vi "WT500 Get Power Data.vi"(7 "Error In":errorcluster, 10 "VISA resource name":refnum<visa-resource-name>) -> (0 "Error Out":errorcluster, 1 "Power Data Out":T1={"Current (A):Element 1"=236.2, "Current (A):Element 2"=17.749, "Power (W):Sigma"=4192.0, "Watt Hours (Wh):Sigma"=0.0, "Voltage (V):Element 2"=236.2, "Voltage (V):Element 1"=236.2, "Current Crest Factor:Element 1"=0.0, "Current Crest Factor:Element 2"=0.0, "Voltage Harmonic (%):Element 1"=0.0, "Voltage Harmonic (%):Element 2"=0.0, "Voltage Crest Factor:Element 1"=0.0, "Voltage Crest Factor:Element 2"=0.0, "Time:Element 1"=0.0, "Frequency (Hz):Element 1"=0.0, "Apparent Power (VA):Element 1"=0.0, "Apparent Power (VA):Element 2"=0.0, "Power Factor:Element 1"=0.0, "Power Factor:Element 2"=0.0, "Max Watt Hours"=0.0, "Voltage (V):Element 2 Avg"=0.0, "Voltage (V):Element 1 Avg"=0.0} {"Voltage (V):Element 1 Avg" format="%.3g"; "Voltage (V):Element 2 Avg" format="%.3g"; "Max Watt Hours" format="%.3g"; "Power Factor:Element 2" format="%.3g"; "Power Factor:Element 1" format="%.3g"; "Apparent Power (VA):Element 2" format="%.3g"; "Apparent Power (VA):Element 1" format="%.3g"; "Frequency (Hz):Element 1" format="%.3g"; "Time:Element 1" format="%.3g"; "Voltage Crest Factor:Element 2" format="%.3g"; "Voltage Crest Factor:Element 1" format="%.3g"; "Voltage Harmonic (%):Element 2" format="%.3g"; "Voltage Harmonic (%):Element 1" format="%.3g"; "Current Crest Factor:Element 2" format="%.3g"; "Current Crest Factor:Element 1" format="%.3g"; "Voltage (V):Element 1" format="%.3g"; "Voltage (V):Element 2" format="%.3g"; "Watt Hours (Wh):Sigma" format="%.3f"; "Power (W):Sigma" format="%.3g"; "Current (A):Element 2" format="%.3e"; "Current (A):Element 1" format="%.3e"}, 2 "Power":dbl, 3 "VISA resource name out":refnum<visa-resource-name>, 4 "Output Array":dbl[](array[numeric]), 6 "Data Array":string[][](array[string]))   [LabVIEW 2019]
uses:
  Trunk/Utility/Type Definitions/UTILITY Power Data.ctl
  LLBs/ykwt500.llb/YKWT500 Read Numeric (Normal).vi
panel:
  in  "Dryer PowerData":T1={"Current (A):Element 1"=236.2, "Current (A):Element 2"=17.749, "Power (W):Sigma"=4192.0, "Watt Hours (Wh):Sigma"=0.0, "Voltage (V):Element 2"=236.2, "Voltage (V):Element 1"=236.2, "Current Crest Factor:Element 1"=0.0, "Current Crest Factor:Element 2"=0.0, "Voltage Harmonic (%):Element 1"=0.0, "Voltage Harmonic (%):Element 2"=0.0, "Voltage Crest Factor:Element 1"=0.0, "Voltage Crest Factor:Element 2"=0.0, "Time:Element 1"=0.0, "Frequency (Hz):Element 1"=0.0, "Apparent Power (VA):Element 1"=0.0, "Apparent Power (VA):Element 2"=0.0, "Power Factor:Element 1"=0.0, "Power Factor:Element 2"=0.0, "Max Watt Hours"=0.0, "Voltage (V):Element 2 Avg"=0.0, "Voltage (V):Element 1 Avg"=0.0} {"Voltage (V):Element 1 Avg" format="%.3g"; "Voltage (V):Element 2 Avg" format="%.3g"; "Max Watt Hours" format="%.3g"; "Power Factor:Element 2" format="%.3g"; "Power Factor:Element 1" format="%.3g"; "Apparent Power (VA):Element 2" format="%.3g"; "Apparent Power (VA):Element 1" format="%.3g"; "Frequency (Hz):Element 1" format="%.3g"; "Time:Element 1" format="%.3g"; "Voltage Crest Factor:Element 2" format="%.3g"; "Voltage Crest Factor:Element 1" format="%.3g"; "Voltage Harmonic (%):Element 2" format="%.3g"; "Voltage Harmonic (%):Element 1" format="%.3g"; "Current Crest Factor:Element 2" format="%.3g"; "Current Crest Factor:Element 1" format="%.3g"; "Voltage (V):Element 1" format="%.3g"; "Voltage (V):Element 2" format="%.3g"; "Watt Hours (Wh):Sigma" format="%.3f"; "Power (W):Sigma" format="%.3g"; "Current (A):Element 2" format="%.3e"; "Current (A):Element 1" format="%.3e"}
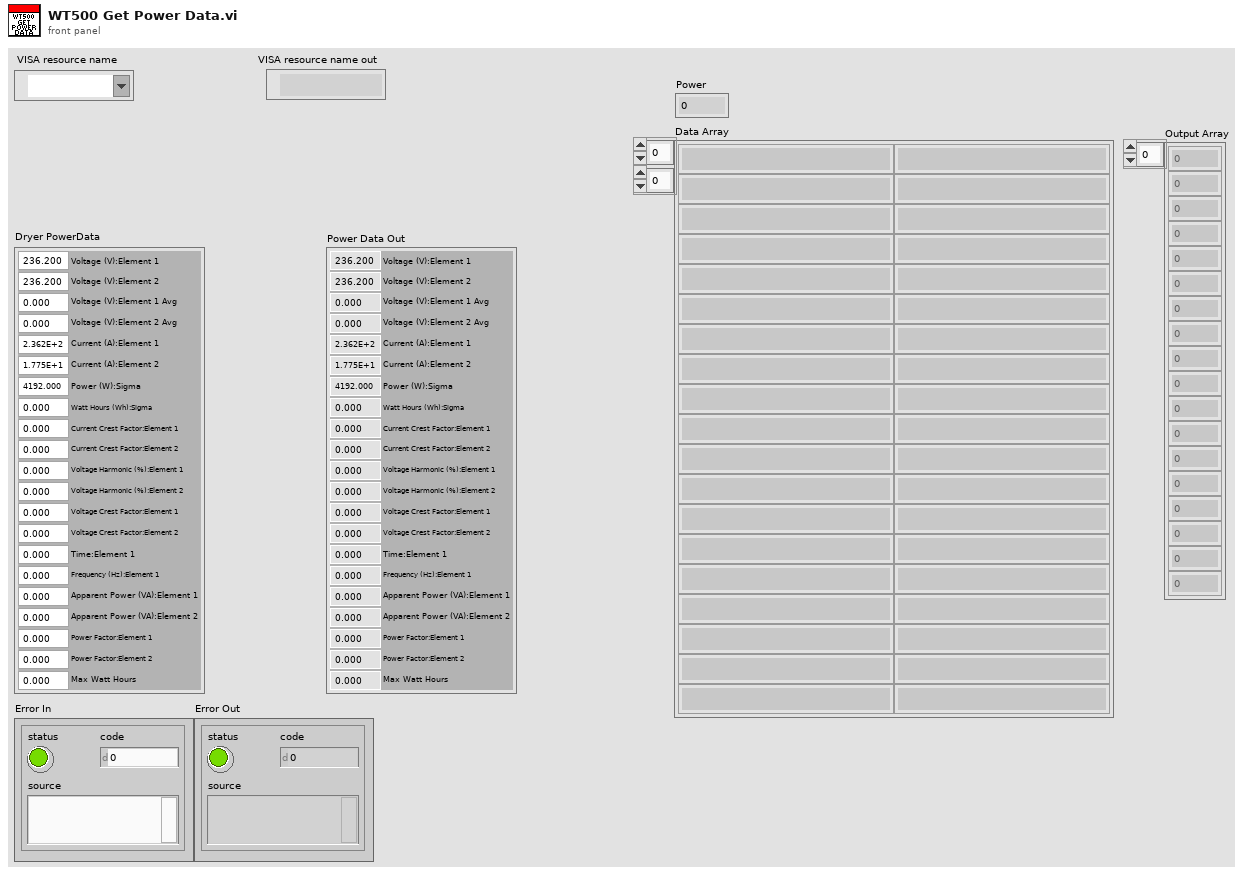
[diagram p1: front panel]
types:
  T1 = typedef "UTILITY Power Data.ctl" = cluster{"Current (A):Element 1":dbl, "Current (A):Element 2":dbl, "Power (W):Sigma":dbl, "Watt Hours (Wh):Sigma":dbl, "Voltage (V):Element 2":dbl, "Voltage (V):Element 1":dbl, "Current Crest Factor:Element 1":dbl, "Current Crest Factor:Element 2":dbl, "Voltage Harmonic (%):Element 1":dbl, "Voltage Harmonic (%):Element 2":dbl, "Voltage Crest Factor:Element 1":dbl, "Voltage Crest Factor:Element 2":dbl, "Time:Element 1":dbl, "Frequency (Hz):Element 1":dbl, "Apparent Power (VA):Element 1":dbl, "Apparent Power (VA):Element 2":dbl, "Power Factor:Element 1":dbl, "Power Factor:Element 2":dbl, "Max Watt Hours":dbl, "Voltage (V):Element 2 Avg":dbl, "Voltage (V):Element 1 Avg":dbl}
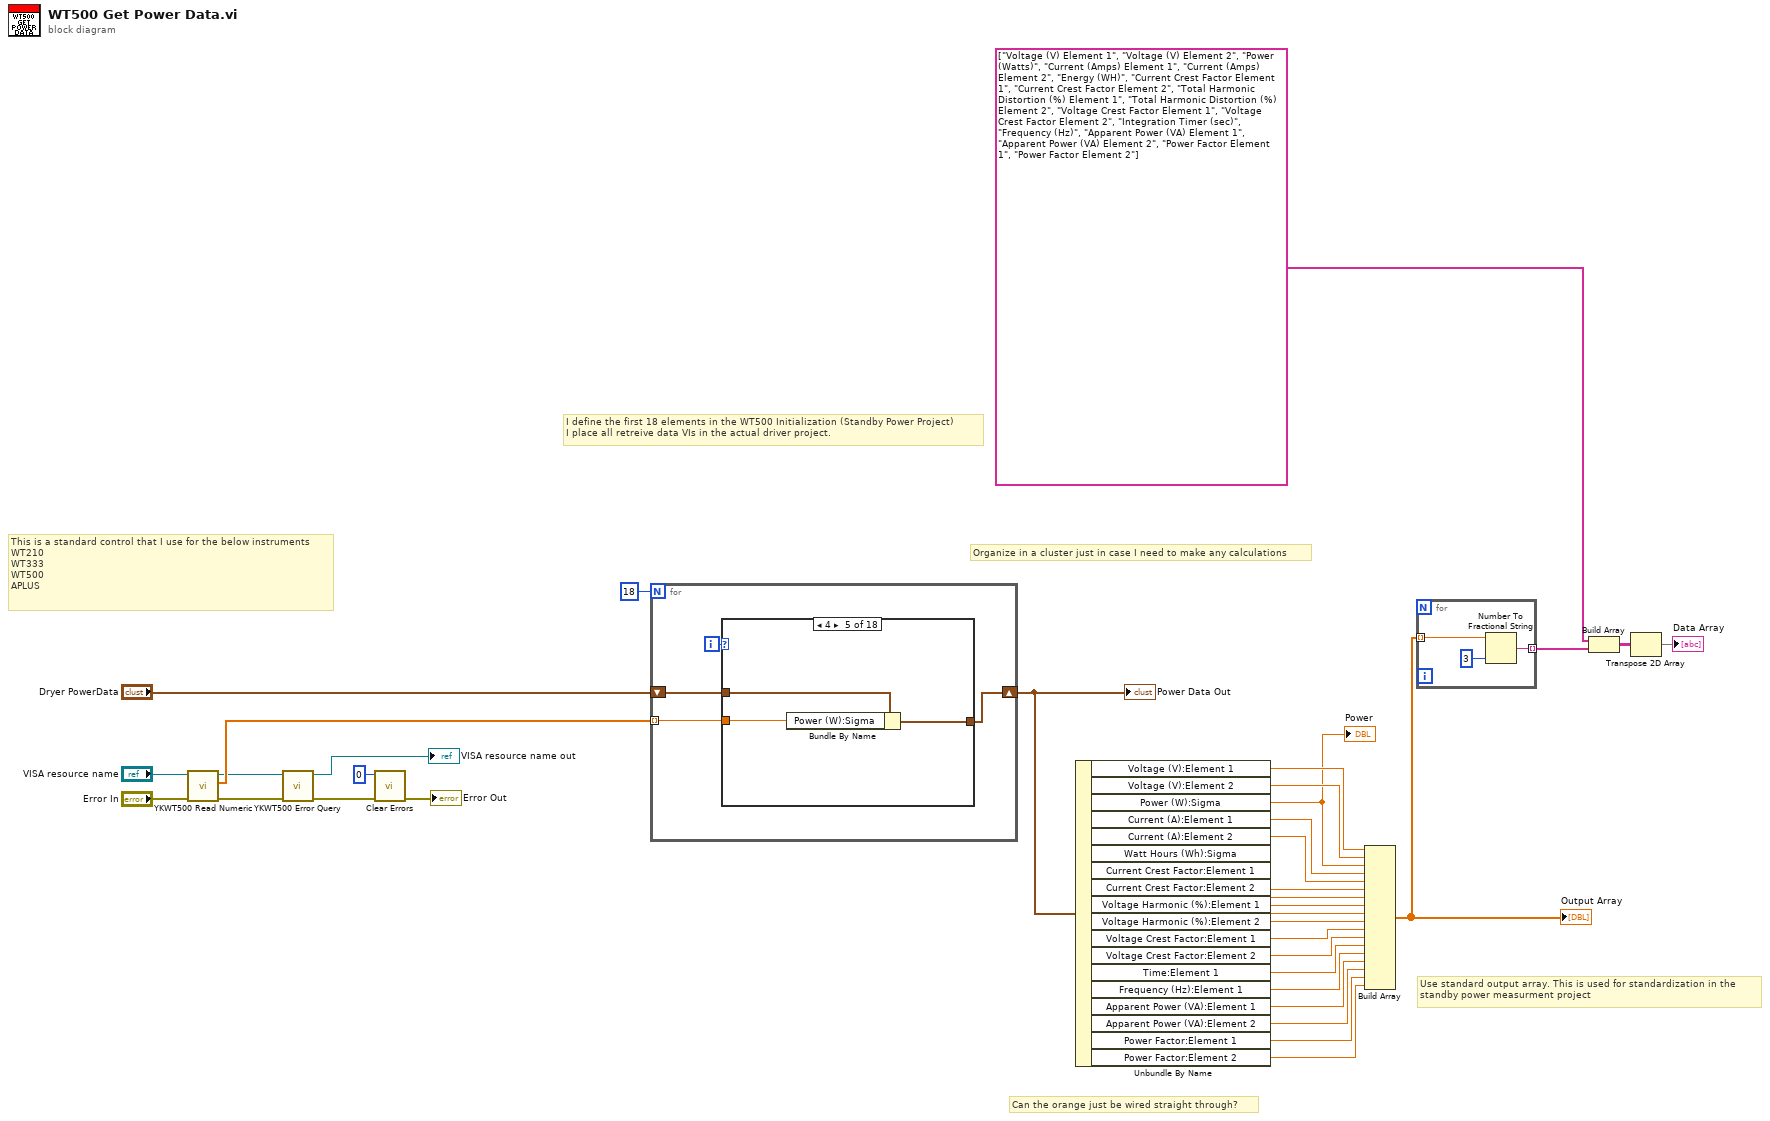
[diagram p0: block diagram]
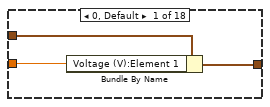
[diagram p2: hidden frame]
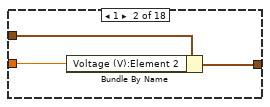
[diagram p3: hidden frame]
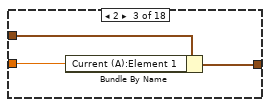
[diagram p4: hidden frame]
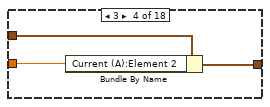
[diagram p5: hidden frame]
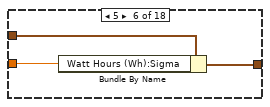
[diagram p6: hidden frame]
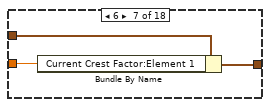
[diagram p7: hidden frame]
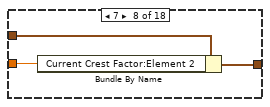
[diagram p8: hidden frame]
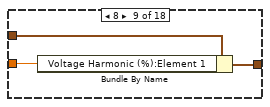
[diagram p9: hidden frame]
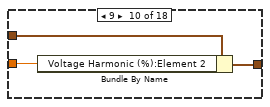
[diagram p10: hidden frame]
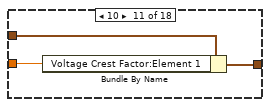
[diagram p11: hidden frame]
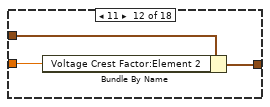
[diagram p12: hidden frame]
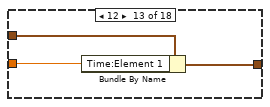
[diagram p13: hidden frame]
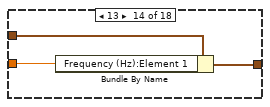
[diagram p14: hidden frame]
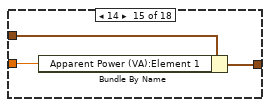
[diagram p15: hidden frame]
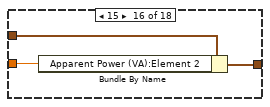
[diagram p16: hidden frame]
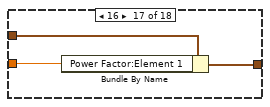
[diagram p17: hidden frame]
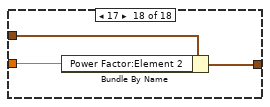
[diagram p18: hidden frame]
diagram:
  # "Can the orange just be wired straight through?"
  # "Use standard output array. This is used for standardization in the \nstandby power measurment project"
  # "Organize in a cluster just in case I need to make any calculations"
  # "This is a standard control that I use for the below instruments\nWT210\nWT333\nWT500\nAPLUS"
  # "I define the first 18 elements in the WT500 Initialization (Standby Power Project)\nI place all retreive data VIs in the actual driver project."
  n1 = call-poly "YKWT500 Read Numeric.vi"("error in (no error)"="Error In", "VISA resource name"="VISA resource name") -> ("error out"=w9:errorcluster, "Measurement Value"=w34:dbl[], "VISA resource name out"=w8:refnum<visa-resource-name>)  [unwired: 7 in]
  n2 = call "YKWT500 Error Query.vi"("error in (no error)"=w9, "VISA resource name"=w8) -> ("error out"=w6:errorcluster, "VISA resource name out"=→"VISA resource name out":refnum<visa-resource-name>)  [unwired: 6 in, 2 out]
  n3 = call <vilib>:"Clear Errors.vi"("error in (no error)"=w6, "specific error code to clear (0: all)"=0) -> ("error out"=→"Error Out":errorcluster)  [unwired: 4 in, 1 out]
  n4 = for {
    N: 18 -> [_]
    tunnel: w34 -> [w36] mode=indexing
    shift-right: [w37] -> w17
    shift-left: "Dryer PowerData" -> [w38]
    i -> [w39]
    n5 = case shown="4" w39 {
      tunnel: w38 -> [w42 w45 w48 w51 w54 w57 w60 w63 w66 w69 w72 w75 w78 w81 w84 w87 w90 w93]
      tunnel: [w41 w44 w47 w50 w53 w56 w59 w62 w65 w68 w71 w74 w77 w80 w83 w86 w89 w92] -> w37
      tunnel: w36 -> [w40 w43 w46 w49 w52 w55 w58 w61 w64 w67 w70 w73 w76 w79 w82 w85 w88 w91]
      frame 0, Default {
        n6 = Bundle By Name(cluster=w42, "Voltage (V):Element 1"=w40) -> (w41:T1)
      }
      frame 1 {
        n7 = Bundle By Name(cluster=w45, "Voltage (V):Element 2"=w43) -> (w44:T1)
      }
      frame 2 {
        n8 = Bundle By Name(cluster=w48, "Current (A):Element 1"=w46) -> (w47:T1)
      }
      frame 3 {
        n9 = Bundle By Name(cluster=w51, "Current (A):Element 2"=w49) -> (w50:T1)
      }
      frame 4 {
        n10 = Bundle By Name(cluster=w54, "Power (W):Sigma"=w52) -> (w53:T1)
      }
      frame 5 {
        n11 = Bundle By Name(cluster=w57, "Watt Hours (Wh):Sigma"=w55) -> (w56:T1)
      }
      frame 6 {
        n12 = Bundle By Name(cluster=w60, "Current Crest Factor:Element 1"=w58) -> (w59:T1)
      }
      frame 7 {
        n13 = Bundle By Name(cluster=w63, "Current Crest Factor:Element 2"=w61) -> (w62:T1)
      }
      frame 8 {
        n14 = Bundle By Name(cluster=w66, "Voltage Harmonic (%):Element 1"=w64) -> (w65:T1)
      }
      frame 9 {
        n15 = Bundle By Name(cluster=w69, "Voltage Harmonic (%):Element 2"=w67) -> (w68:T1)
      }
      frame 10 {
        n16 = Bundle By Name(cluster=w72, "Voltage Crest Factor:Element 1"=w70) -> (w71:T1)
      }
      frame 11 {
        n17 = Bundle By Name(cluster=w75, "Voltage Crest Factor:Element 2"=w73) -> (w74:T1)
      }
      frame 12 {
        n18 = Bundle By Name(cluster=w78, "Time:Element 1"=w76) -> (w77:T1)
      }
      frame 13 {
        n19 = Bundle By Name(cluster=w81, "Frequency (Hz):Element 1"=w79) -> (w80:T1)
      }
      frame 14 {
        n20 = Bundle By Name(cluster=w84, "Apparent Power (VA):Element 1"=w82) -> (w83:T1)
      }
      frame 15 {
        n21 = Bundle By Name(cluster=w87, "Apparent Power (VA):Element 2"=w85) -> (w86:T1)
      }
      frame 16 {
        n22 = Bundle By Name(cluster=w90, "Power Factor:Element 1"=w88) -> (w89:T1)
      }
      frame 17 {
        n23 = Bundle By Name(cluster=w93, "Power Factor:Element 2"=w91) -> (w92:T1)
      }
    }
  }
  "Power Data Out" <- w17
  n24 = Unbundle By Name(w17) -> ("Voltage (V):Element 1"=w18:dbl, "Voltage (V):Element 2"=w19:dbl, "Power (W):Sigma"=w1:dbl, "Current (A):Element 1"=w2:dbl, "Current (A):Element 2"=w3:dbl, "Watt Hours (Wh):Sigma"=w11:dbl, "Current Crest Factor:Element 1"=w20:dbl, "Current Crest Factor:Element 2"=w21:dbl, "Voltage Harmonic (%):Element 1"=w22:dbl, "Voltage Harmonic (%):Element 2"=w23:dbl, "Voltage Crest Factor:Element 1"=w24:dbl, "Voltage Crest Factor:Element 2"=w25:dbl, "Time:Element 1"=w26:dbl, "Frequency (Hz):Element 1"=w27:dbl, "Apparent Power (VA):Element 1"=w28:dbl, "Apparent Power (VA):Element 2"=w29:dbl, "Power Factor:Element 1"=w30:dbl, "Power Factor:Element 2"=w31:dbl)
  "Power" <- w1
  n25 = Build Array(w18, w19, w1, w2, w3, w11, w20, w21, w22, w23, w24, w25, w26, w27, w28, w29, w30, w31) -> (w16:dbl[])
  "Output Array" <- w16
  n26 = for {
    tunnel: w16 -> [w96] mode=indexing
    tunnel: [w94] -> w14 mode=indexing
    n27 = Number To Fractional String(number=w96, precision (6)=i16 3) -> (F-format string=w94:string)  [unwired: 2 in]
  }
  n28 = Build Array(string[] ["Voltage (V) Element 1", "Voltage (V) Element 2", "Power (Watts)", "Current (Amps) Element 1", "Current (Amps) Element 2", "Energy (WH)", "Current Crest Factor Element 1", "Current Crest Factor Element 2", "Total Harmonic Distortion (%) Element 1", "Total Harmonic Distortion (%) Element 2", "Voltage Crest Factor Element 1", "Voltage Crest Factor Element 2", "Integration Timer (sec)", "Frequency (Hz)", "Apparent Power (VA) Element 1", "Apparent Power (VA) Element 2", "Power Factor Element 1", "Power Factor Element 2"], w14) -> (w13:string[][])
  n29 = Transpose 2D Array(2D array=w13) -> (transposed array=→"Data Array":string[][])
